vi "Actor Core.vi"(8 "error in":errorcluster, 11 "HIJ Vision Fluence Cam Launcher in":refnum<class "HIJ Vision Fluence Cam Launcher.lvclass">) -> (0 "error out":errorcluster, 3 "Actor out":refnum<class "Actor.lvclass">)   [LabVIEW 2014, in "HIJ Vision Fluence Cam.lvlib" / "HIJ Vision Fluence Cam Launcher.lvclass"]
doc: "(<B>Filename</B>: Actor Framework.lvlib:Actor.lvclass:Actor Core.vi)\n\nReceives messages to the actor, reacts to them, and initiates any error handling that may shut the actor down.\n\nDescendant classes may override this VI to append parallel tasks for the actor to complete while it handles messages. Overrides use the Call Parent Method node."
uses:
  HIJ Vision Fluence Cam Launcher.lvclass
  <vilib>/ActorFramework/Actor/Actor.lvclass
  HIJ Vision Launcher/HIJ Vision Launcher/HIJ Vision Launcher.lvclass/HIJ Vision Launcher.ctl
  <vilib>/ActorFramework/Actor/Actor.lvclass/Actor.ctl
  <vilib>/ActorFramework/Message Enqueuer/Message Enqueuer.lvclass/Message Enqueuer.ctl
  HIJ Vision Fluence Cam/HIJ Vision Fluence Cam.lvclass
  HIJ Vision Fluence Cam/HIJ Vision Fluence Cam.lvclass/HIJ Vision Fluence Cam.ctl
  HIJ Vision Fluence Cam Launcher Messages/Set F Start Parameter Msg/Set F Start Parameter Msg.lvclass/Set F Start Parameter Msg.ctl
  HIJ Vision Fluence Cam/Write @Energy.vi
  HIJ Vision Fluence Cam/Write Size of Region.vi
  HIJ Vision Launcher/HIJ Vision Launcher/Read HIJ Vision Camera App.vi
  HIJ Vision Launcher/HIJ Vision Launcher/Write HIJ Vision Camera App.vi
  <vilib>/ActorFramework/Message Enqueuer/Init from Existing Queue.vi
  <vilib>/ActorFramework/Message Enqueuer/Enqueue.vi
  <vilib>/Utility/config.llb/Read Key (U32).vi
  <vilib>/Utility/config.llb/Read Key (Double).vi
  <vilib>/Utility/config.llb/Write Key (U32).vi
  <vilib>/Utility/config.llb/Write Key (Double).vi
  <vilib>/ActorFramework/Message Priority Queue/Priority Enqueue.vi
  Viewable Actor/ViewableActor/ViewableActor.lvclass
  <vilib>/ActorFramework/Message Enqueuer/Message Enqueuer.lvclass
  HIJ Vision Fluence Cam Launcher Messages/Set F Start Parameter Msg/Set F Start Parameter Msg.lvclass
  <vilib>/ActorFramework/Stop Msg/Stop Msg.lvclass
  HIJ Vision Launcher/HIJ Vision Launcher/HIJ Vision Launcher.lvclass
  <vilib>/Utility/config.llb/NI_LVConfig.lvlib
panel:
  in  "Stop":bool=TRUE
  in  "@Energy":dbl[unit]=10.0 format="%#_13g"
  in  "Size of Region":u8=2
  # "px"
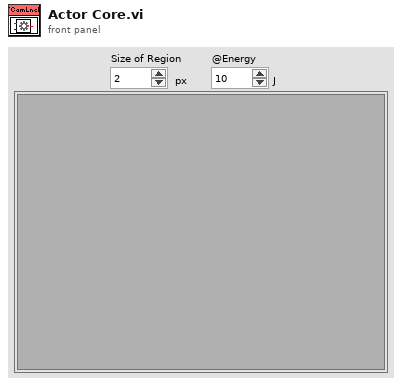
[diagram p1: front panel]
types:
  T1 = typedef "NI_LVConfig.lvlib/Config Data RefNum.ctl" = refnum<k1>
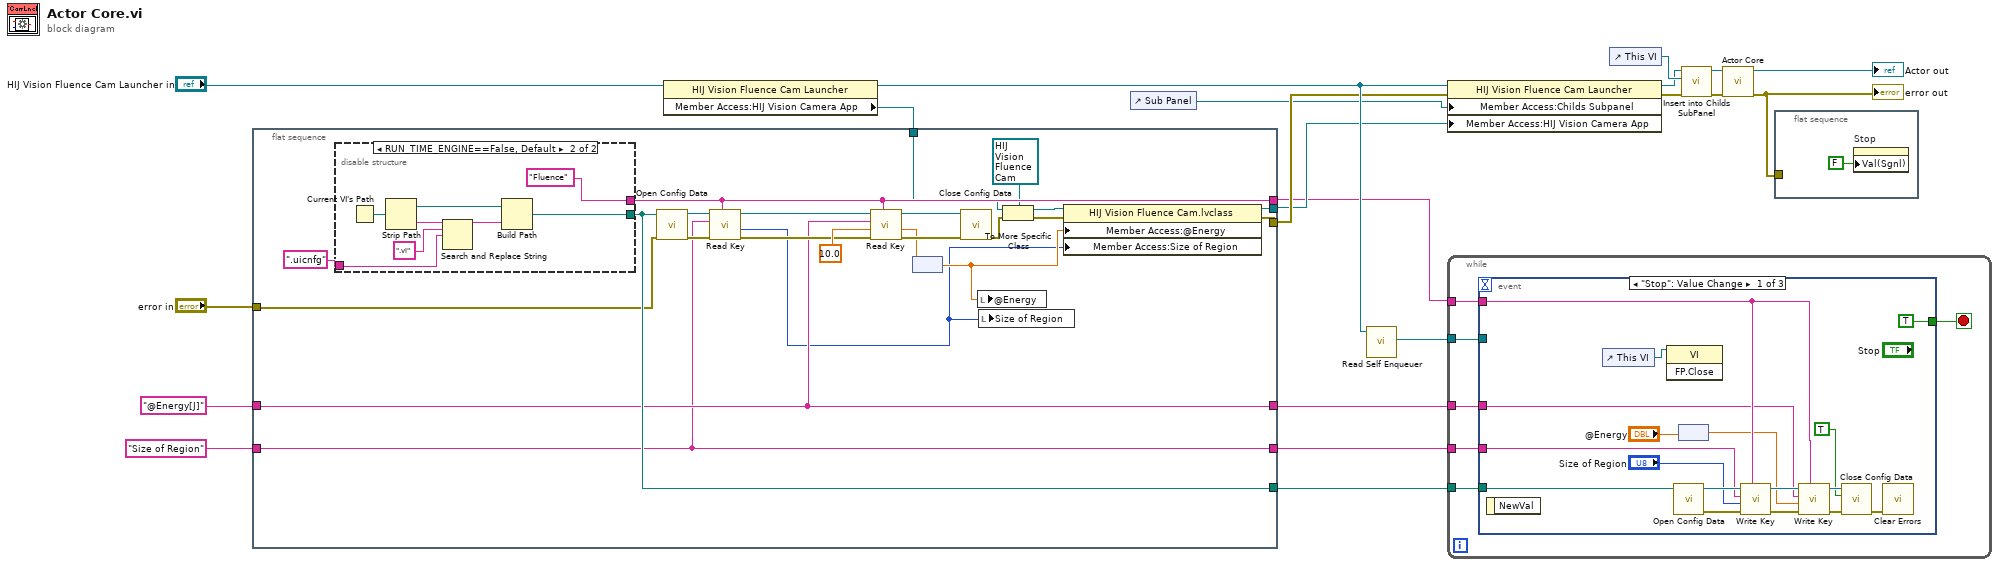
[diagram p0: block diagram]
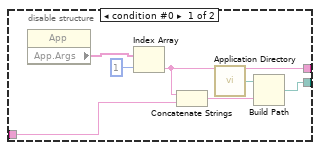
[diagram p2: hidden frame]
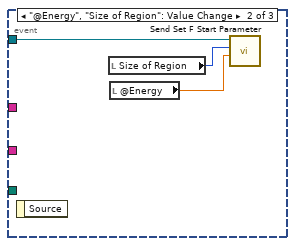
[diagram p3: hidden frame]
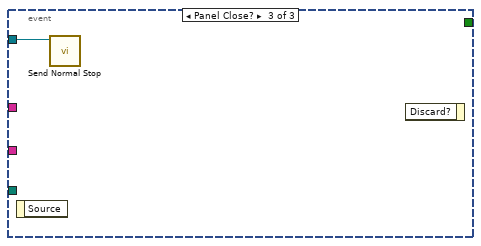
[diagram p4: hidden frame]
diagram:
  n1 = flat-sequence {
    tunnel: [w37] -> w12
    tunnel: [w36] -> w11
    tunnel: "@Energy[J]" ("key") -> [w30]
    tunnel: "Size of Region" ("key") -> [w29]
    tunnel: [w35] -> w9
    tunnel: "error in" -> [w32]
    tunnel: [w31] -> w20
    tunnel: [w30] -> w6
    tunnel: [w29] -> w4
    tunnel: w3 -> [w24]
    frame #0 {
      n2 = disable-structure shown="RUN_TIME_ENGINE==False, Default" {
        disable-tunnel: [w47 w53] -> w37
        disable-tunnel: ".uicnfg" ("string") -> [w46 w56]
        disable-tunnel: [w45 "Fluence"] -> w35
        frame condition #0 {
          n3 = property class="App"() -> ("App.Args"=w51:string[])  [unwired: 2 in, 2 out]
          n4 = Index Array(array=w51, index=1) -> (element=w45:string)
          n5 = Concatenate Strings(w45, w46) -> (w48:string)
          n6 = call <vilib>:"Application Directory.vi"() -> ("Application Directory"=w49:path)
          n7 = Build Path(base path=w49, name or relative path=w48) -> (appended path=w47:path)
        }
        frame condition #1 (active) {
          n8 = Current VI's Path() -> (path=w59:path)
          n9 = Strip Path(path=w59) -> (stripped path=w54:path, name=w58:string)
          n10 = Search and Replace String(input string=w58, search string=".vi", replace string=w56) -> (result string=w55:string)  [unwired: 5 in, 3 out]
          n11 = Build Path(base path=w54, name or relative path=w55) -> (appended path=w53:path)
        }
      }
      n12 = call <vilib>:"Open Config Data.vi"("error in (no error)"=w32, "configuration file path"=w37) -> ("error out"=w43:errorcluster, "refnum"=w42:T1)  [unwired: 7 in, 1 out]
      n13 = call-poly <vilib>:"Read Key.vi"("section"=w35, "error in (no error)"=w43, "key"=w29, "refnum"=w42) -> ("error out"=w34:errorcluster, "value"=w27:u32, "refnum out"=w41:T1)  [unwired: 4 in, 1 out]
      n14 = call-poly <vilib>:"Read Key.vi"("section"=w35, "error in (no error)"=w34, "default value"=10.0 ("@Energy"), "key"=w30, "refnum"=w41) -> ("error out"=w33:errorcluster, "value"=w28:dbl, "refnum out"=w40:T1)  [unwired: 3 in, 1 out]
      n15 = node(w28) -> (w38:dbl[unit])
      n16 = call <vilib>:"Close Config Data.vi"("error in (no error)"=w33, "refnum"=w40) -> ("error out"=w23:errorcluster)  [unwired: 8 in, 1 out]
      n17 = local write "@Energy"(w38) -> ()
      n18 = local write "Size of Region"(w27) -> ()
      n19 = To More Specific Class(target class=refnum<class "HIJ Vision Fluence Cam.lvclass"> refnum ("HIJ Vision Fluence Cam.lvlib:HIJ Vision Fluence Cam.lvclass"), reference=w24, error in=w23) -> (specific class reference=w26:refnum<class "HIJ Vision Fluence Cam.lvclass">, error out=w22:errorcluster)
      n20 = property class="HIJ Vision Fluence Cam.lvclass"(reference=w26, error in=w22, "Member Access:@Energy"=w38, "Member Access:Size of Region"=w27) -> (reference out=w36:refnum<class "HIJ Vision Fluence Cam.lvclass">, error out=w31:errorcluster)
    }
  }
  n21 = property class="HIJ Vision Fluence Cam Launcher"(reference="HIJ Vision Fluence Cam Launcher in") -> (reference out=w21:refnum<class "HIJ Vision Fluence Cam Launcher.lvclass">, "Member Access:HIJ Vision Camera App"=w3:refnum<class "ViewableActor.lvclass">)  [unwired: 1 in, 1 out]
  n22 = control-ref of="Sub Panel"() -> (w18:refnum<vi>)
  n23 = call <vilib>:"Read Self Enqueuer.vi"("Actor"=w21) -> ("Self Enqueuer"=w1:refnum<class "Message Enqueuer.lvclass">)  [unwired: 10 in]
  n24 = property class="HIJ Vision Fluence Cam Launcher"(reference=w21, error in=w20, "Member Access:Childs Subpanel"=w18, "Member Access:HIJ Vision Camera App"=w11) -> (reference out=w2:refnum<class "HIJ Vision Fluence Cam Launcher.lvclass">, error out=w7:errorcluster)
  n25 = while {
    tunnel: w12 -> [w65]
    tunnel: w6 -> [w64]
    tunnel: w4 -> [w63]
    tunnel: w9 -> [w61]
    tunnel: w1 -> [w60]
    stop <- w62 stop-if-true
    n26 = event shown="[0] \"Stop\": Value Change" {
      selector: _ -> [_ _ _]
      dyn-events: _ -> [_ _ _]
      timeout: _ -> [_ _ _]
      tunnel: w65 -> [w73 _ _]
      tunnel: w64 -> [w72 _ _]
      tunnel: w63 -> [w71 _ _]
      tunnel: [TRUE _ _] -> w62
      tunnel: w61 -> [w82 _ _]
      tunnel: w60 -> [_ w85 w86]
      event "Stop": Value Change {
        n27 = event-data() -> ()  [unwired: 1 in, 1 out]
        n28 = control-ref of="This VI"() -> (w66:refnum<vi>)
        n29 = invoke class="VI" method="FP.Close"(reference=w66) -> ()  [unwired: 2 in, 3 out]
        n30 = call <vilib>:"Open Config Data.vi"("configuration file path"=w73) -> ("error out"=w75:errorcluster, "refnum"=w74:T1)  [unwired: 8 in, 1 out]
        n31 = node("@Energy") -> (w68:dbl)
        n32 = call-poly <vilib>:"Write Key.vi"("section"=w82, "error in (no error)"=w75, "value"="Size of Region", "key"=w71, "refnum"=w74) -> ("error out"=w80:errorcluster, "refnum out"=w78:T1)  [unwired: 4 in, 1 out]
        n33 = call-poly <vilib>:"Write Key.vi"("section"=w82, "error in (no error)"=w80, "value"=w68, "key"=w72, "refnum"=w78) -> ("error out"=w81:errorcluster, "refnum out"=w79:T1)  [unwired: 4 in, 1 out]
        n34 = call <vilib>:"Close Config Data.vi"("error in (no error)"=w81, "write file if changed (T)"=TRUE, "refnum"=w79) -> ("error out"=w76:errorcluster)  [unwired: 7 in, 1 out]
        n35 = call <vilib>:"Clear Errors.vi"("error in (no error)"=w76) -> ()  [unwired: 5 in, 2 out]
      }
      event "@Energy", "Size of Region": Value Change {
        n36 = event-data() -> ()  [unwired: 1 in, 1 out]
        n37 = local read "Size of Region"() -> (w84:u8)
        n38 = local read "@Energy"() -> (w83:dbl[unit])
        n39 = call "Send Set F Start Parameter.vi"("@Energy"=w83, "Size of Region"=w84, "Message Enqueuer"=w85) -> ()  [unwired: 7 in, 2 out]
      }
      event Panel Close? {
        n40 = event-data() -> ()  [unwired: 1 in, 1 out]
        n41 = call <vilib>:"Send Normal Stop.vi"("Message Enqueuer"=w86) -> ()  [unwired: 10 in, 1 out]
        n42 = event-data() -> ()  [unwired: 2 in, 1 out]
      }
    }
  }
  n43 = control-ref of="This VI"() -> (w14:refnum<vi>)
  n44 = call-dynamic "Insert into Childs SubPanel.vi"("error in (no error)"=w7, "UI VI Ref"=w14, "ViewableActorEncaps in"=w2) -> ("error out"=w15:errorcluster, "ViewableActorEncaps out"=w16:refnum<class "HIJ Vision Fluence Cam Launcher.lvclass">)  [unwired: 7 in]
  n45 = call-parent "Actor Core.vi"("error in"=w15, "HIJ Vision Launcher in"=w16) -> ("error out"=w13:errorcluster, "Actor out"=→"Actor out":refnum<class "Actor.lvclass">)  [unwired: 8 in]
  "error out" <- w13
  n46 = flat-sequence {
    tunnel: w13 -> [_]
    frame #0 {
      n47 = property on="Stop" class="Bool (strict)"("Val(Sgnl)"=FALSE ("Value (Signaling)")) -> ()  [unwired: 2 in, 2 out]
    }
  }
